vi "Upload File.vi"(6 "Chunk size (kB)":i32=5120 min=5120, 8 "error in (no error)":errorcluster, 9 "Object Path (including file name)":string, 10 "file to upload":path, 11 "Data.S3":refnum<class "Data.S3.lvclass">) -> (0 "error out":errorcluster, 3 "Data.S3":refnum<class "Data.S3.lvclass">)   [LabVIEW 2020, in "Data.S3.lvclass"]
uses:
  Data.S3.lvclass
  Data.S3.lvclass/Data.S3.ctl
  <vilib>/AWS Toolkit/S3/Bucket/Bucket.lvclass
panel:
  # "* an object path includes the name of the file, and does not include\nthe bucket name. e.g:\nPPMS2/SA03008N.20190801/031_sideGateSweep.tdms"
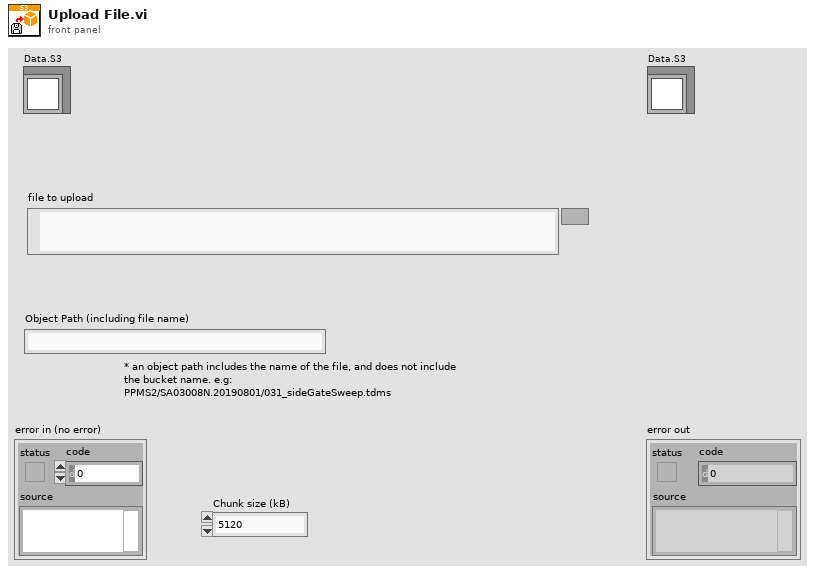
[diagram p1: front panel]
types:
  T1 = typedef "NI_AWS_Core.lvlib/HTTP Request.lvclass/AWS Credentials.ctl" = cluster{"Access Key":string, "Secret Key":string}
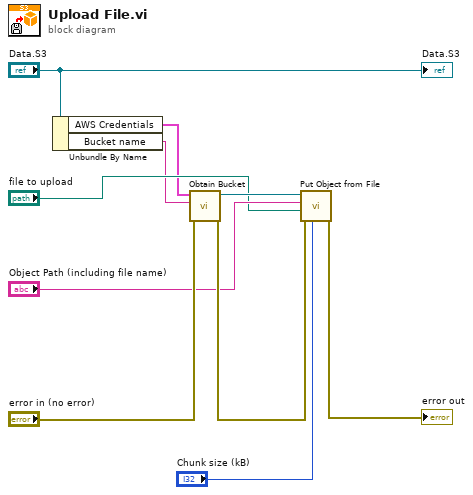
[diagram p0: block diagram]
diagram:
  n1 = Unbundle By Name("Data.S3") -> ("AWS Credentials"=w3:T1, "Bucket name"=w2:string)
  n2 = call <vilib>:"Obtain Bucket.vi"("error in (no error)"="error in (no error)", "Bucket name"=w2, "AWS Credentials"=w3) -> ("error out"=w9:errorcluster, "Bucket"=w8:refnum<class "Bucket.lvclass">)  [unwired: 7 in]
  n3 = call <vilib>:"Put Object from File.vi"("Chunk size (kB)"="Chunk size (kB)", "error in (no error)"=w9, "File"="file to upload", "Object Path"="Object Path (including file name)", "Bucket in"=w8) -> ("error out"=→"error out":errorcluster)  [unwired: 2 in, 4 out]
  "Data.S3" <- "Data.S3"
